vi "GetDisplayName.vi"(8 "error in (no error)":errorcluster, 11 "CGrapherDGML in":refnum<class "CGrapherDGML.lvclass">) -> (0 "error out":errorcluster, 1 "Display name":string, 3 "CGrapherDGML out":refnum<class "CGrapherDGML.lvclass">)   [LabVIEW 2020, in "DefaultExtensions.lvlib" / "CGrapherDGML.lvclass"]
uses:
  CGrapherDGML.lvclass
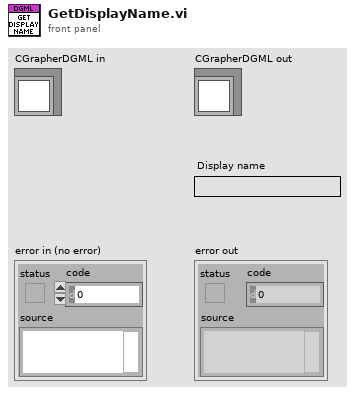
[diagram p1: front panel]
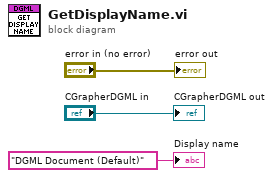
[diagram p0: block diagram]
diagram:
  "error out" <- "error in (no error)"
  "CGrapherDGML out" <- "CGrapherDGML in"
  "Display name" <- "DGML Document (Default)" ("Display name")
